vi "Dat2TDMS.vi"(8 "error in (no error)":errorcluster, 11 "file path":path) -> (0 "error out":errorcluster)   [LabVIEW 2018]
uses:
  <vilib>/Utility/file.llb/Read From Spreadsheet File (string).vi
panel:
  in  "Cancel Button":bool
  out "Progress":dbl(slide) scale=0.0..1.0
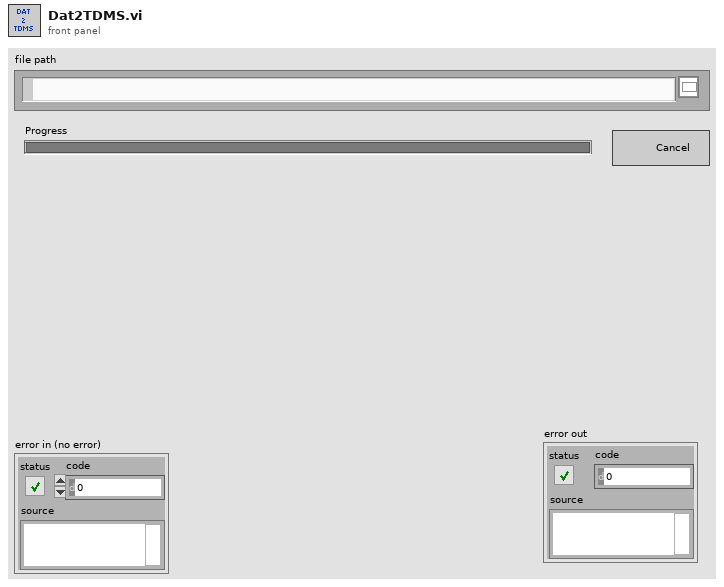
[diagram p1: front panel]
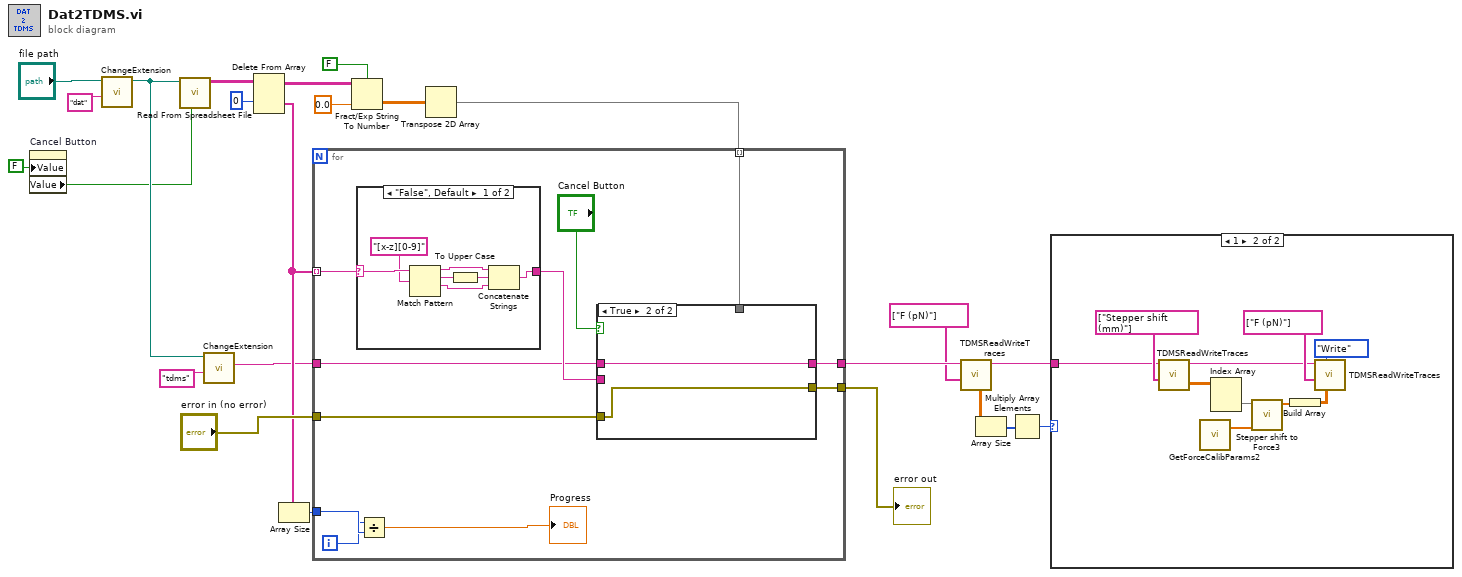
[diagram p0: block diagram]
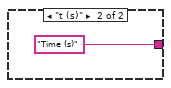
[diagram p3: hidden frame]
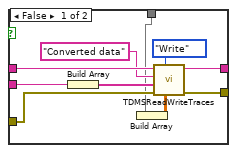
[diagram p4: hidden frame]
diagram:
  n1 = property on="Cancel Button" class="Bool (strict)"("Value"=FALSE ("Cancel Button")) -> ("Value"=w8:bool)  [unwired: 2 in, 2 out]
  n2 = call "ChangeExtension.vi"("extension"="dat", "Path in"="file path") -> ("Path out"=w15:path)  [unwired: 3 in, 4 out]
  n3 = call-poly <vilib>:"Read From Spreadsheet File.vi"("transpose (no:F)"=w8, "file path (dialog if empty)"=w15) -> ("all rows"=w23:string[][])  [unwired: 5 in, 4 out]
  n4 = call "ChangeExtension.vi"("extension"="tdms", "Path in"=w15) -> ("file out"=w7:string)  [unwired: 3 in, 4 out]
  n5 = Delete From Array(array=w23, index (row)=0) -> (deleted portion=w11:string[], array with subset deleted=w21:string[][])  [unwired: 2 in]
  n6 = Array Size(array=w11) -> (size(s)=w10:i32)
  n7 = Fract/Exp String To Number(use system decimal point (T)=FALSE, string=w21, default (0 dbl)=0.0 ("default (0 DBL)")) -> (number=w19:dbl[][])  [unwired: 1 in, 1 out]
  n8 = Transpose 2D Array(2D array=w19) -> (transposed array=w14:dbl[][])
  n9 = for {
    tunnel: w14 -> [w35] mode=indexing
    tunnel: w11 -> [w28] mode=indexing
    tunnel: "error in (no error)" -> [w34]
    tunnel: [w33] -> w12
    tunnel: w10 -> [w31]
    tunnel: w7 -> [w26]
    tunnel: [w25] -> w6
    i -> [w30]
    n10 = case shown="\"False\", Default" w28 {
      selector: w28 -> [w42 _]
      tunnel: [w37 "Time (s)"] -> w27
      frame "False", Default {
        n11 = Match Pattern(string=w42, regular expression="[x-z][0-9]" ("format string")) -> (before substring=w36:string, match substring=w40:string, after substring=w38:string)  [unwired: 1 in, 1 out]
        n12 = To Upper Case(1:w40) -> (0:w39:string)
        n13 = Concatenate Strings(w36, w39, w38) -> (w37:string)
      }
      frame "t (s)" {
      }
    }
    n14 = Divide(x=w30, y=w31) -> (x/y=→"Progress":dbl)
    n15 = case shown="True" "Cancel Button" {
      tunnel: w35 -> [w47 _]
      tunnel: w27 -> [w53 _]
      tunnel: w34 -> [w51 w55]
      tunnel: [w52 w55] -> w33
      tunnel: w26 -> [w50 w54]
      tunnel: [w44 w54] -> w25
      frame False {
        n16 = Build Array(w53) -> (w49:string[])
        n17 = Build Array(w47) -> (w46:dbl[][])
        n18 = call "TDMSReadWriteTraces.vi"("Data in"=w46, "Task"=enum16{"Read", "Write"}."Write", "error in (no error)"=w51, "Channels in"=w49, "group name"="Converted data", "tracename"=w50) -> ("error out"=w52:errorcluster, "tracename out"=w44:string)  [unwired: 4 out]
      }
      frame True {
      }
    }
  }
  "error out" <- w12
  n19 = call "TDMSReadWriteTraces.vi"("Channels in"=string[] ["F (pN)"], "tracename"=w6) -> ("tracename out"=w5:string, "Data out"=w3:dbl[][])  [unwired: 4 in, 4 out]
  n20 = Array Size(array=w3) -> (size(s)=w1:i32[])
  n21 = Multiply Array Elements(1:w1) -> (0:w2:i32)
  n22 = case shown="1" w2 {
    tunnel: w5 -> [_ w57]
    frame 0, Default {
    }
    frame 1 {
      n23 = call "TDMSReadWriteTraces.vi"("Channels in"=string[] ["Stepper shift (mm)"], "tracename"=w57) -> ("tracename out"=w56:string, "Data out"=w65:dbl[][])  [unwired: 4 in, 4 out]
      n24 = call "GetForceCalibParams2.vi"() -> ("F1/L1/F0/F2/L2"=w64:dbl[])  [unwired: 6 in, 1 out]
      n25 = Index Array(array=w65) -> (element=w62:dbl[])  [unwired: 2 in]
      n26 = call "Stepper shift to Force3.vi"("F1/L1/F0/F2/L2"=w64, "Stepper Shift"=w62) -> ("Force(pN)"=w59:dbl[])  [unwired: 4 in, 1 out]
      n27 = Build Array(w59) -> (w60:dbl[][])
      n28 = call "TDMSReadWriteTraces.vi"("Data in"=w60, "Task"=enum16{"Read", "Write"}."Write", "Channels in"=string[] ["F (pN)"], "tracename"=w56) -> ()  [unwired: 2 in, 6 out]
    }
  }
